vi "1.5.9-Extraction.vi"(0 "Block Memory":refnum<k21>="Multiplier 1 Block Memory Out : [8b Identifier; 6b args; 18b fxp output]", 1 "Watched Channel":u8, 2 "Count to match":u8, 3 "Writing Index Start":u32, 4 "Timeout":i32=120) -> (5 "Writing Index End":u32, 6 "Timed out":bool, 7 "Multiplication Result":fxp<+/-,18,1> format="%.18g")   [LabVIEW 2010]
uses:
  <vilib>/Platform/TimedLoop/XDataNode/XDataNode.xnode
  <vilib>/Platform/TimedLoop/XDataNode/timing_clust.ctl
  <vilib>/Platform/TimedLoop/XDataNode/nitl_modes.ctl
  <vilib>/Platform/TimedLoop/XDataNode/wakeup.ctl
  <vilib>/rvi/DataTransferAndStorage/Container/XNode/niFpgaContainer.xnode
  <vilib>/rvi/DataTransferAndStorage/Container/Common/niFpgaContainerMetaDataKey.ctl
  1.0-Hindbrain Global.vi
  <vilib>/rvi/DataTransferAndStorage/Container/Common/niFpgaContainerExecOnDevCompGetState.vi
  <vilib>/rvi/Memory/Memory_Emulation/nirvimemoryEmulationManagerCache_GetValue.vi
  <vilib>/rvi/DataTransferAndStorage/Container/Common/niFpgaContainerGetUniqueNameForEmu.vi
  <vilib>/rvi/Memory/Memory_Emulation/nirvimemoryEmulationManagerCache_InsertValue.vi
  <vilib>/Utility/error.llb/Clear Errors.vi
  <vilib>/Platform/TimedLoop/XDataNode/XDNodeRunTimeDep.lvlib
  <vilib>/rvi/Memory/Memory_Emulation/nirvimemoryEmulationManagerCache_SetValue.vi
panel:
  out "Writing Index After the best one":u32
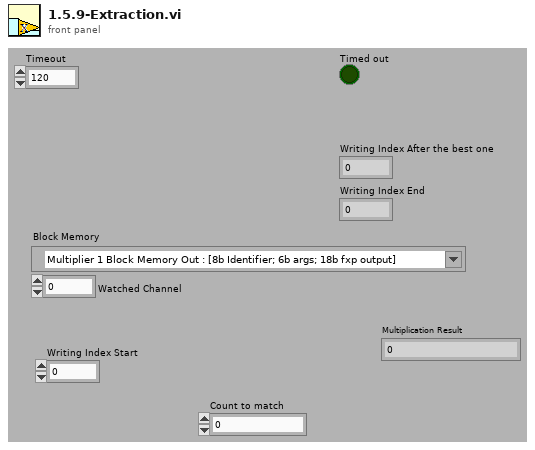
[diagram p1: front panel]
types:
  T1 = typedef "XDNodeRunTimeDep.lvlib/timing_clust.ctl" = cluster{"Expected End [f-1]":u64, "Actual End [f-1]":u64, "Finished Late? [f-1]":bool, "Expected End [i-1]":u64, "Actual End [i-1]":u64, "Finished Late? [i-1]":bool, "Expected Start [i]":u64, "Actual Start [i]":u64, "Expected Start [f]":u64, "Actual Start [f]":u64, "Source Name":string, "Structure Name":string, "Period":i64, "Deadline":i64, "Offset":i64, "Start":i64, "Priority":i32, "Timeout":i32, "Mode":T2, "Wakeup Reason":T3, "Error":errorcluster, "Source Type":string, "Secondary Source Type":string, "Global End Time":u64, "Global Start Time":u64, "Frame Duration":u64, "Iteration Duration":u64, "Assigned CPU":i32, "I/O Scan Engine Mode":u32}
  T2 = typedef "XDNodeRunTimeDep.lvlib/nitl_modes.ctl" = enum32{"No Change", "Process missed periods, maintain original phase", "Discard missed periods, maintain original phase", "Process missed periods, ignore original phase", "Discard missed periods, ignore original phase"}
  T3 = typedef "XDNodeRunTimeDep.lvlib/wakeup.ctl" = enum32{"Normal", "Aborted", "Asynchronous wakeup", "Timing source error", "Timed loop error", "Timeout"}
  T4 = typedef "niFpgaContainerMetaDataKey.ctl" = enum16{"FPGA FIFO", "FPGA Memory", "FPGA Register"}
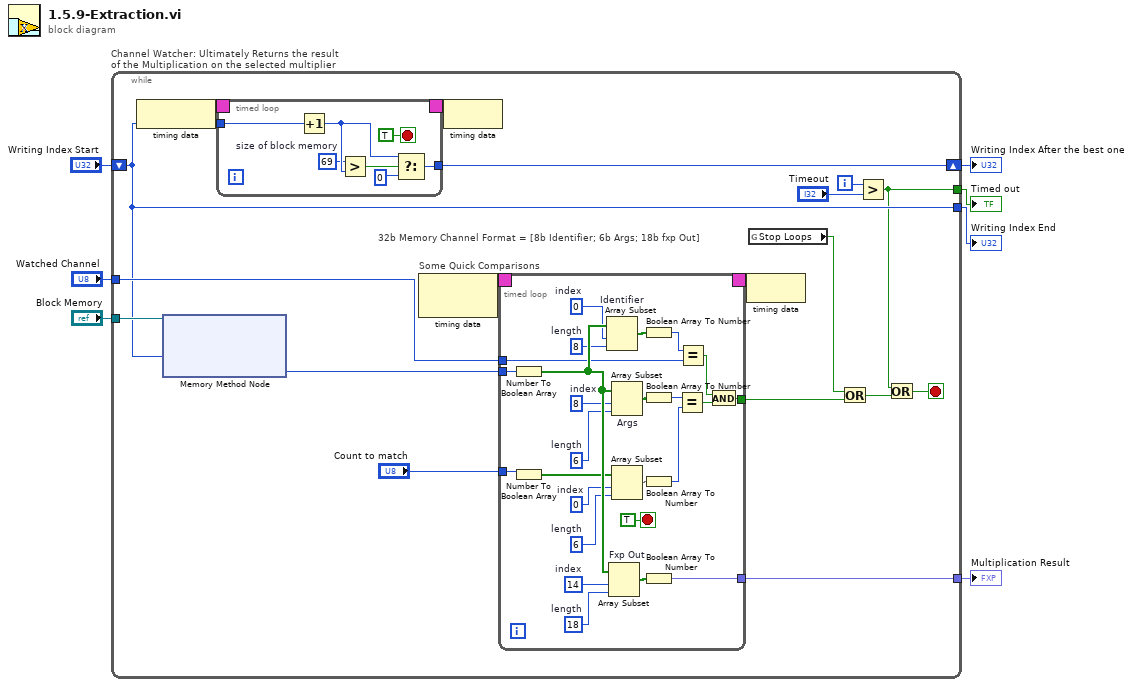
[diagram p0: block diagram]
diagram:
  n1 = while "Channel Watcher: Ultimately Returns the result of the Multiplication on the selected multiplier" {
    shift-right: [w17] -> w3
    shift-left: "Writing Index Start" -> [w14]
    tunnel: "Watched Channel" -> [w22]
    tunnel: "Block Memory" -> [w21]
    tunnel: [w20] -> w4
    tunnel: [w14] -> w2
    tunnel: [w10] -> w1
    i -> [w12]
    stop <- w11 stop-if-true
    # "32b Memory Channel Format = [8b Identifier; 6b Args; 18b fxp Out]"
    n2 = node-c288() -> (w16:T1)
    n3 = xnode ("Memory Method Node")("Address"=w14, "Memory In"=w21) -> ("Data"=w25:u32)  [unwired: 1 out]
    n4 = timed-loop {
      timing: w16 -> [_]
      timing-out: [_] -> w15
      tunnel: w14 -> [w28]
      tunnel: [w27] -> w17
      stop <- TRUE stop-if-true
      w30 = u32 69  # size of block memory
      n5 = Increment(x=w28) -> (x+1=w31:u32)
      n6 = Greater?(x=w30, y=w31) -> (0:w29:bool)
      n7 = Select(t=w31, s=w29, f=u32 0) -> (s? t:f=w27:u32)
    }
    n8 = node-c288() -> (w24:T1)  [unwired: 1 in]
    n9 = node-c288(w15) -> ()
    n10 = timed-loop "Some Quick Comparisons" {
      timing: w24 -> [_]
      timing-out: [_] -> w23
      tunnel: w25 -> [w50]
      tunnel: w22 -> [w49]
      tunnel: [w48] -> w20
      tunnel: [w47] -> w18
      tunnel: "Count to match" -> [w37]
      stop <- TRUE stop-if-true
      w41 = 6  # length
      w42 = 0  # index
      w55 = 8  # length
      w56 = 6  # length
      w57 = 18  # length
      w58 = 14  # index
      w59 = 8  # index
      w60 = 0  # index
      n11 = Number To Boolean Array(number=w50) -> (Boolean array=w61:bool[])
      n12 = Number To Boolean Array(number=w37) -> (Boolean array=w44:bool[])
      n13 = Array Subset "Identifier"(array=w61, index=w60, length=w55) -> (w54:bool[])
      n14 = Array Subset "Fxp Out"(array=w61, index=w58, length=w57) -> (w53:bool[])
      n15 = Array Subset "Args"(array=w61, index=w59, length=w56) -> (w45:bool[])
      n16 = Array Subset(array=w44, index=w42, length=w41) -> (w43:bool[])
      n17 = Boolean Array To Number(Boolean array=w54) -> (number=w52:u8)
      n18 = Boolean Array To Number(Boolean array=w45) -> (number=w40:u8)
      n19 = Boolean Array To Number(Boolean array=w43) -> (number=w39:u8)
      n20 = Boolean Array To Number(Boolean array=w53) -> (number=w48:fxp<+/-,18,1>)
      n21 = Equal?(x=w40, y=w39) -> (x = y?=w38:bool)
      n22 = Equal?(x=w52, y=w49) -> (x = y?=w51:bool)
      n23 = And ("We have what we want")(x=w51, y=w38) -> (x .and. y?=w47:bool)
    }
    n24 = node-c288(w23) -> ()
    n25 = global read "1.0-Hindbrain Global.vi" "Stop Loops"() -> (w9:bool)
    n26 = Or(x=w9, y=w18) -> (x .or. y?=w19:bool)
    n27 = Greater?(x=w12, y="Timeout") -> (0:w10:bool)
    n28 = Or(x=w10, y=w19) -> (x .or. y?=w11:bool)
  }
  "Multiplication Result" <- w4
  "Writing Index After the best one" <- w3
  "Writing Index End" <- w2
  "Timed out" <- w1
